vi "Write DebuggingTerminal.vi"(10 "DebuggingTerminal":refnum<class "DebuggingTerminal.lvclass">, 11 "Connection in":refnum<class "Connection.lvclass">) -> (3 "Connection out":refnum<class "Connection.lvclass">)   [LabVIEW 2013, in "MQTT_Connection.lvlib" / "Connection.lvclass"]
uses:
  Connection.lvclass
  MQTT_Base/DebuggingTerminal/DebuggingTerminal.lvclass
  Connection.lvclass/Connection.ctl
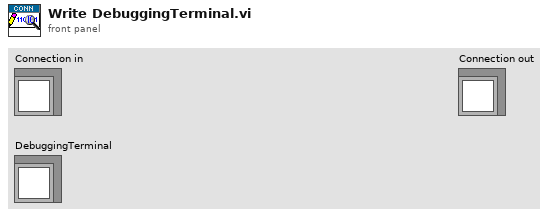
[diagram p1: front panel]
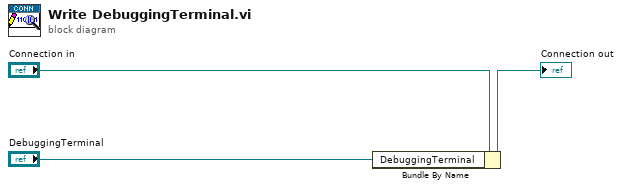
[diagram p0: block diagram]
diagram:
  n1 = Bundle By Name(cluster="Connection in", "DebuggingTerminal"="DebuggingTerminal") -> (→"Connection out":refnum<class "Connection.lvclass">)
